vi "Get Certificate Count.vi"(8 "error in (no error)":errorcluster, 10 "buffer size":u32, 11 "store":string) -> (0 "error out":errorcluster, 3 "count":u32)   [LabVIEW 2020, in "CodeSignAPI.lvlib"]
doc: "getcertinfo(const char *store, char *buff, unsigned int bufsize);"
uses:
  <vilib>/AppBuilder/CodeSignAPI/CodeSignAPI.lvlib
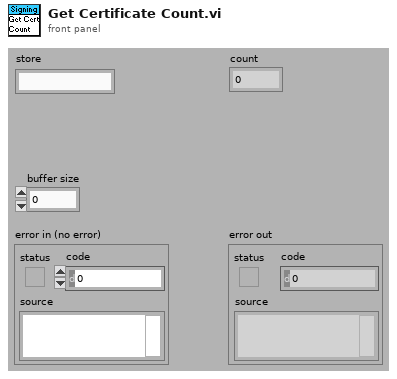
[diagram p1: front panel]
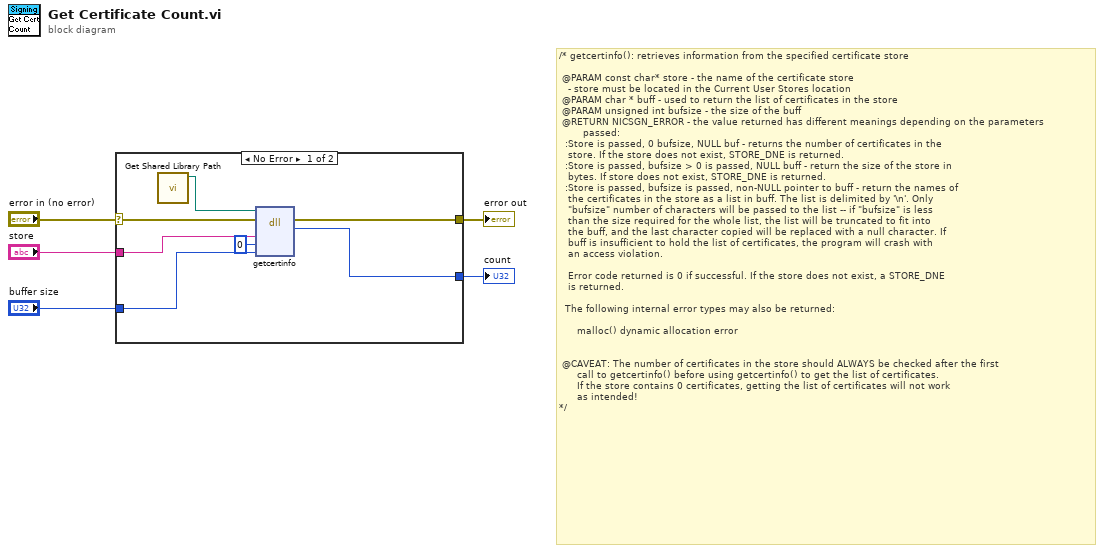
[diagram p0: block diagram]
diagram:
  # "/* getcertinfo(): retrieves information from the specified certificate store\n\n\t@PARAM const char* store - the name of the certificate store\n\t\t\t- store must be located in the Current User Stores location\n\t@PARAM char * buff - used to return the list of certificates in the store\n\t@PARAM unsigned int bufsize - the size of the buff\n\t@RETURN NICSGN_ERROR - the value returned has different meanings depending on the parameters\n\t\t\t\t\t\t\t\tpassed:\n\t\t:Store is passed, 0 bufsize, NULL buf - returns the number of certificates in the\n\t\t\tstore. If the store does not exist, STORE_DNE is returned.\n\t\t:Store is passed, bufsize > 0 is passed, NULL buff - return the size of the store in\n\t\t\tbytes. If store does not exist, STORE_DNE is returned.\n\t\t:Store is passed, bufsize is passed, non-NULL pointer to buff - return the names of\n\t\t\tthe certificates in the store as a list in buff. The list is delimited by '\\n'. Only\n\t\t\t\"bufsize\" number of characters will be passed to the list -- if \"bufsize\" is less\n\t\t\tthan the size required for the whole list, the list will be truncated to fit into\n\t\t\tthe buff, and the last character copied will be replaced with a null character. If\n\t\t\tbuff is insufficient to hold the list of certificates, the program will crash with\n\t\t\tan access violation.\n\n\t\t\tError code returned is 0 if successful. If the store does not exist, a STORE_DNE \n\t\t\tis returned.\n\n\t\tThe following internal error types may also be returned: \n\t\t\t\n      malloc() dynamic allocation error\n\n\n\t@CAVEAT: The number of certificates in the store should ALWAYS be checked after the first\n      call to getcertinfo() before using getcertinfo() to get\tthe list of certificates.\n      If the store contains 0 certificates, getting the list of certificates will not work\n      as intended!\n*/"
  n1 = case shown="No Error" "error in (no error)" {
    selector: "error in (no error)" -> [w9 w13]
    tunnel: [w8 _] -> w5
    tunnel: "store" -> [w12 _]
    tunnel: "buffer size" -> [w11 _]
    tunnel: [w7 w13] -> w2
    frame No Error {
      n2 = call <vilib>:"Get Shared Library Path.vi"() -> ("shared library path"=w10:path)  [unwired: 1 in, 10 out]
      n3 = dll-call lib="?" fn="getcertinfo"(path in=w10, error in=w9, "store"=w12, "buff"=u64 0, "bufsize"=w11) -> (error out=w7:errorcluster, "return type"=w8:i64)  [unwired: 3 in, 2 out]
    }
    frame Error {
    }
  }
  "count" <- w5
  "error out" <- w2
